vi "Begin.vi"   [LabVIEW 2016]
doc: "Called before other user functions, this VI is expected to open initial I/O refnums, load in file data, and do all program initialization. Notice that the <B>error out</B> terminal is simply used for data flow. Wiring it to other structures or subVIs ensures that this VI runs first."
uses:
  <vilib>/Rock Robotics/SystemInterfaces/DIO/FPGA_DIOPWMChannel.ctl
  <vilib>/Rock Robotics/WPI/Joystick/WPI_JoystickDeviceEnum.ctl
  <vilib>/Rock Robotics/WPI/SafetyOutput/WPI_SafetyOutputConfigMenu.ctl
  <vilib>/Rock Robotics/WPI/RobotDrive/WPI_RobotDriveOpen4MotorWithVictorSP.vi
  <vilib>/Rock Robotics/WPI/MotorControl/WPI_MotorControlOpen VictorSP.vi
  External/2ndContollerStatus.vi
  <vilib>/Rock Robotics/WPI/RobotDrive/WPI_RobotDriveOpen2MotorWithVictorSP.vi
types:
  T1 = typedef "FPGA_DIOPWMChannel.ctl" = enum8{"PWM 0", "PWM 1", "PWM 2", "PWM 3", "PWM 4", "PWM 5", "PWM 6", "PWM 7", "PWM 8", "PWM 9", "PWM MXP 0", "PWM MXP 1", "PWM MXP 2", "PWM MXP 3", "PWM MXP 4", "PWM MXP 5", "PWM MXP 6", "PWM MXP 7", "PWM MXP 8", "PWM MXP 9", "Invalid"}
  T2 = typedef "WPI_SafetyOutputConfigMenu.ctl" = enum16{"Enable", "Disable"}
  T3 = typedef "WPI_JoystickDeviceEnum.ctl" = enum16{"USB 0", "USB 1", "USB 2", "USB 3", "USB 4", "USB 5"}
  T4 = typedef "WPI_JoystickDevRef.ctl" = cluster{"Device":T3}
  T5 = typedef "WPI_ServoDeviceRef.ctl" = cluster{"DeviceStatus":errorcluster, "PWM Channel":T1, "DeadBand":T6}
  T6 = typedef "WPI_PWMDeadband.ctl" = cluster{"Name":string, "maxPositivePwm":i32, "minPositivePwm":i32, "centerPwm":i32, "maxNegativePwm":i32, "minNegativePwm":i32, "angularRange":u16}
  T7 = typedef "WPI_MotorControlDeviceRef.ctl" = cluster{"DeviceStatus":errorcluster, "Type":T8, "PWM":cluster{"PWM Channel":T1, "DeadBand":T6}, "CAN":cluster{"Device Number":u8, "SetOutput VI Ref":variant, "GetOutput VI Ref":variant, "Enable VI Ref":variant, "Disable VI Ref":variant, "Data":variant}, "Invert":bool}
  T8 = typedef "WPI_MotorControlType.ctl" = enum16{"PWM", "CAN"}
  T9 = typedef "WPI_RobotDriveDevRef.ctl" = cluster{"DevStatus":errorcluster, "Motors[]":T7[], "Square Inputs":bool, "Max Output":dbl}
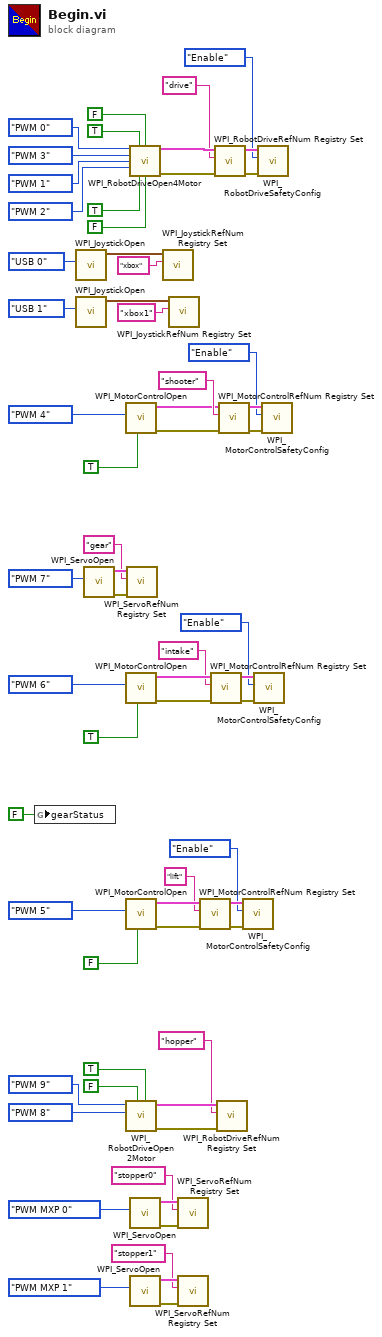
[diagram p0: block diagram]
diagram:
  n1 = global write "2ndContollerStatus.vi" "gearStatus"(FALSE ("gearStatus")) -> ()
  n2 = call <vilib>:"WPI_JoystickOpen.vi"("JoystickDevice"=WPI_JoystickDeviceEnum."USB 0") -> ("JoystickDevRef"=w53:T4)  [unwired: 10 in]
  n3 = call <vilib>:"WPI_JoystickOpen.vi"("JoystickDevice"=WPI_JoystickDeviceEnum."USB 1") -> ("JoystickDevRef"=w27:T4)  [unwired: 10 in]
  n4 = call <vilib>:"WPI_ServoOpen.vi"("PWM Channel"=FPGA_DIOPWMChannel."PWM 7") -> ("error out"=w41:errorcluster, "ServoDeviceRef"=w42:T5)  [unwired: 9 in]
  n5 = call-poly <vilib>:"WPI_MotorControlOpen.vi"("Invert"=TRUE, "PWM Channel"=FPGA_DIOPWMChannel."PWM 4") -> ("error out"=w45:errorcluster, "MotorControlDeviceRef"=w46:T7)  [unwired: 8 in]
  n6 = call-poly <vilib>:"WPI_MotorControlOpen.vi"("Invert"=TRUE, "PWM Channel"=FPGA_DIOPWMChannel."PWM 6") -> ("error out"=w34:errorcluster, "MotorControlDeviceRef"=w35:T7)  [unwired: 8 in]
  n7 = call-poly <vilib>:"WPI_MotorControlOpen.vi"("Invert"=FALSE, "PWM Channel"=FPGA_DIOPWMChannel."PWM 5") -> ("error out"=w22:errorcluster, "MotorControlDeviceRef"=w23:T7)  [unwired: 8 in]
  n8 = call-poly <vilib>:"WPI_RobotDriveOpen2Motor.vi"("Right Motor Inverted"=TRUE, "Left Motor Inverted"=FALSE, "Right Motor"=FPGA_DIOPWMChannel."PWM 8" ("PWM Channel"), "Left Motor"=FPGA_DIOPWMChannel."PWM 9") -> ("error out"=w13:errorcluster, "RobotDriveDevRef"=w14:T9)  [unwired: 6 in]
  n9 = call <vilib>:"WPI_ServoRefNum Registry Set.vi"("error in (no error)"=w41, "refnum name"="gear", "ServoDeviceRef"=w42) -> ()  [unwired: 7 in, 2 out]
  n10 = call-poly <vilib>:"WPI_RobotDriveOpen4Motor.vi"("Rear Left Motor"=FPGA_DIOPWMChannel."PWM 0", "Rear Left Motor Inverted"=TRUE, "Rear Right Motor Inverted"=FALSE, "Rear Right Motor"=FPGA_DIOPWMChannel."PWM 3", "Front Left Motor"=FPGA_DIOPWMChannel."PWM 1", "Front Right Motor"=FPGA_DIOPWMChannel."PWM 2", "Front Left Motor Inverted"=TRUE, "Front Right Motor Inverted"=FALSE) -> ("RobotDriveDevRef"=w60:T9, "error out"=w59:errorcluster)  [unwired: 6 in]
  n11 = call <vilib>:"WPI_ServoOpen.vi"("PWM Channel"=FPGA_DIOPWMChannel."PWM MXP 0") -> ("error out"=w6:errorcluster, "ServoDeviceRef"=w7:T5)  [unwired: 9 in]
  n12 = call <vilib>:"WPI_ServoOpen.vi"("PWM Channel"=FPGA_DIOPWMChannel."PWM MXP 1") -> ("error out"=w2:errorcluster, "ServoDeviceRef"=w3:T5)  [unwired: 9 in]
  n13 = call <vilib>:"WPI_JoystickRefNum Registry Set.vi"("refnum name"="xbox", "JoystickDevRef"=w53) -> ()  [unwired: 8 in, 2 out]
  n14 = call <vilib>:"WPI_JoystickRefNum Registry Set.vi"("refnum name"="xbox1", "JoystickDevRef"=w27) -> ()  [unwired: 8 in, 2 out]
  n15 = call <vilib>:"WPI_ServoRefNum Registry Set.vi"("error in (no error)"=w6, "refnum name"="stopper0", "ServoDeviceRef"=w7) -> ()  [unwired: 7 in, 2 out]
  n16 = call <vilib>:"WPI_ServoRefNum Registry Set.vi"("error in (no error)"=w2, "refnum name"="stopper1", "ServoDeviceRef"=w3) -> ()  [unwired: 7 in, 2 out]
  n17 = call <vilib>:"WPI_MotorControlRefNum Registry Set.vi"("error in (no error)"=w22, "refnum name"="lift", "MotorControlDevRef"=w23) -> ("error out"=w19:errorcluster, "MotorControlDevRef"=w20:T7)  [unwired: 7 in]
  n18 = call <vilib>:"WPI_MotorControlRefNum Registry Set.vi"("error in (no error)"=w34, "refnum name"="intake", "MotorControlDevRef"=w35) -> ("error out"=w31:errorcluster, "MotorControlDevRef"=w32:T7)  [unwired: 7 in]
  n19 = call <vilib>:"WPI_RobotDriveRefNum Registry Set.vi"("error in (no error)"=w59, "refnum name"="drive", "RobotDriveDevRef"=w60) -> ("error out"=w56:errorcluster, "RobotDriveDevRef"=w57:T9)  [unwired: 7 in]
  n20 = call <vilib>:"WPI_RobotDriveRefNum Registry Set.vi"("error in (no error)"=w13, "refnum name"="hopper", "RobotDriveDevRef"=w14) -> ()  [unwired: 7 in, 2 out]
  n21 = call <vilib>:"WPI_MotorControlRefNum Registry Set.vi"("error in (no error)"=w45, "refnum name"="shooter", "MotorControlDevRef"=w46) -> ("error out"=w38:errorcluster, "MotorControlDevRef"=w39:T7)  [unwired: 7 in]
  n22 = call <vilib>:"WPI_MotorControlSafetyConfig.vi"("error in (no error)"=w19, "mode"=WPI_SafetyOutputConfigMenu."Enable", "MotorControlDevRef"=w20) -> ()  [unwired: 7 in, 2 out]
  n23 = call <vilib>:"WPI_MotorControlSafetyConfig.vi"("error in (no error)"=w31, "mode"=WPI_SafetyOutputConfigMenu."Enable", "MotorControlDevRef"=w32) -> ()  [unwired: 7 in, 2 out]
  n24 = call <vilib>:"WPI_RobotDriveSafetyConfig.vi"("error in (no error)"=w56, "mode"=WPI_SafetyOutputConfigMenu."Enable", "RobotDriveDevRef"=w57) -> ()  [unwired: 7 in, 2 out]
  n25 = call <vilib>:"WPI_MotorControlSafetyConfig.vi"("error in (no error)"=w38, "mode"=WPI_SafetyOutputConfigMenu."Enable", "MotorControlDevRef"=w39) -> ()  [unwired: 7 in, 2 out]
